vi "Disable Live Comm.vi"(8 "error in (no error)":errorcluster, 11 "TEC 1090 in":refnum<class "Meerstetter TEC.lvclass">) -> (0 "error out":errorcluster, 3 "TEC 1090 out":refnum<class "Meerstetter TEC.lvclass">)   [LabVIEW 2015, in "Meerstetter Lib.lvlib" / "Meerstetter TEC.lvclass"]
uses:
  Meerstetter TEC.lvclass
  reusable/Session APIs/Serial/Serial Session.lvclass
  Meerstetter TEC.lvclass/Meerstetter TEC.ctl
  Configurable Device/Configurable Device.lvclass/Configurable Device.ctl
  Accessors/Read SerialSession.vi
  Configurable Device/Read Log Session.vi
  Configurable Device/Read ID.vi
  reusable/Session APIs/Serial/Public/Asynchronous Write.vi
  reusable/Session APIs/Serial/Public/Asynchronous Read.vi
  <vilib>/MSR Consulting, LLC/ESF/Session - Root.lvclass
  reusable/Session APIs/Session Log/System Log.lvclass
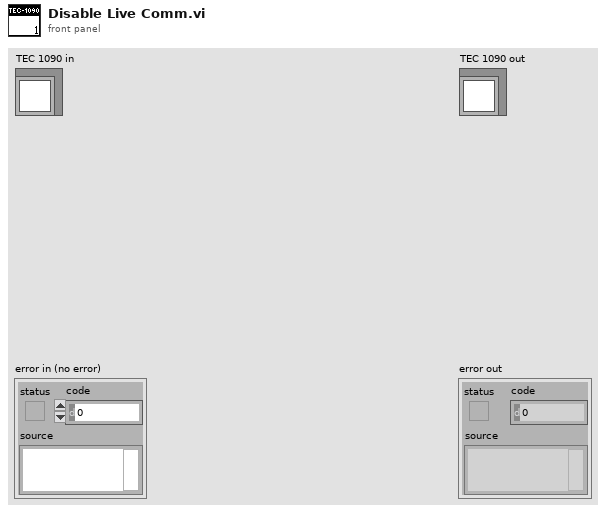
[diagram p1: front panel]
types:
  T1 = typedef "Session - Root.lvclass/Session Handle.ctl" = refnum<data-value>
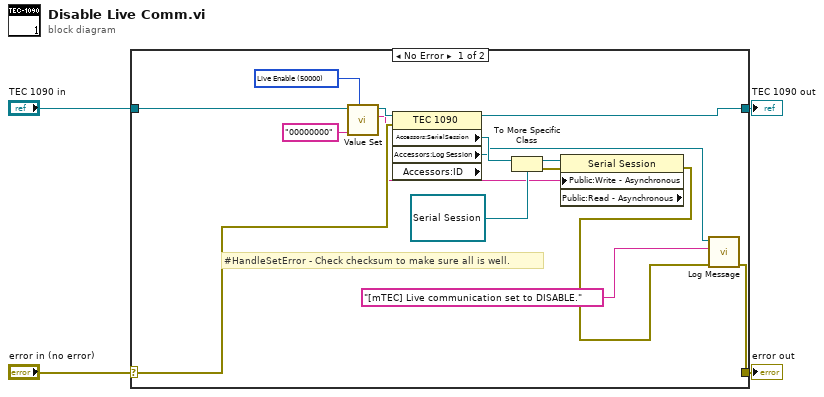
[diagram p0: block diagram]
diagram:
  n1 = case shown="No Error" "error in (no error)" {
    selector: "error in (no error)" -> [w16 w21]
    tunnel: [w8 w21] -> w3
    tunnel: [w11 w20] -> w1
    tunnel: "TEC 1090 in" -> [w19 w20]
    frame No Error {
      w18 = u16 50000 items=["Input Selection"=2000, "Status"=2010, "Set Current"=2020, "Set Voltage"=2021, "Current Limitation"=2030, "Voltage Limitation"=2031, "Current Error Threshold"=2032, "Voltage Error Threshold"=2033, "Channel Baud Rate"=2050, "Response Delay"=2052, "Timeout"=2060, "Target Object Temperature"=3000, "Coarse Temp Ramp"=3003, "Proximity Width"=3002, "Kp"=3010, "Ti"=3011, "Td"=3012, "D Part Damping D1"=3013, "Live Enable"=50000, "Live Set Current"=50001, "Live Set Voltage"=50002, "Object Target Temperature"=50012, "Save Data to Flash"=108] ("Value Set")
      # "#HandleSetError - Check checksum to make sure all is well."
      n2 = call "Value Set.vi"("Value Set"=w18, "Value"="00000000", "TEC 1090"=w19) -> ("hex integer string"=w10:string, "TEC 1091"=w17:refnum<class "Meerstetter TEC.lvclass">)  [unwired: 7 in]
      n3 = property class="TEC 1090" props=["Accessors:SerialSession", "Accessors:Log Session", "Accessors:ID"](reference=w17, error in=w16) -> (reference out=w11:refnum<class "Meerstetter TEC.lvclass">, "Accessors:SerialSession"=w15:T1, "Accessors:Log Session"=w9:T1)  [unwired: 2 out]
      n4 = To More Specific Class(target class=refnum<data-value> refnum, reference=w15) -> (specific class reference=w13:refnum<data-value>, error out=w12:errorcluster)  [unwired: 1 in]
      n5 = property class="Serial Session" props=["Public:Write - Asynchronous", "Public:Read - Asynchronous"](reference=w13, error in=w12, "Public:Write - Asynchronous"=w10) -> (error out=w6:errorcluster)  [unwired: 2 out]
      n6 = call "Log Message.vi"("error in"=w6, "MSG In"="[mTEC] Live communication set to DISABLE." ("format string"), "session in"=w9) -> ("error out"=w8:errorcluster)  [unwired: 7 in, 1 out]
    }
    frame Error {
    }
  }
  "error out" <- w3
  "TEC 1090 out" <- w1
